vi "SPIDelaySet.vi"(8 "error in (no error)":errorcluster caption="错误输入（无错误）", 10 "Delay(CLK)":i32(ring) items=["0"=0, "1"=1, "2"=2, "5"=5, "10"=10, "20"=20], 11 "handle":u64) -> (0 "error out":errorcluster caption="错误输出", 2 "function return":i32, 3 "handle out":u64)   [LabVIEW 2018]
doc: "Set pos. or neg. Supply voltage"
uses:
  InstrumentsPlayground.lvlib
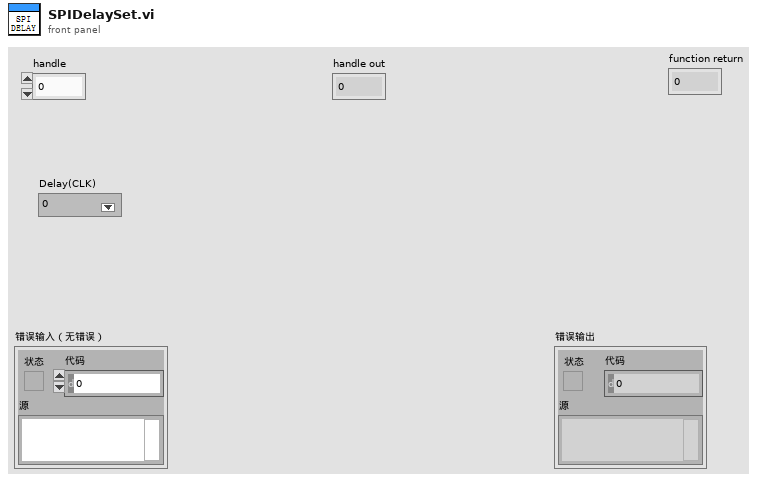
[diagram p1: front panel]
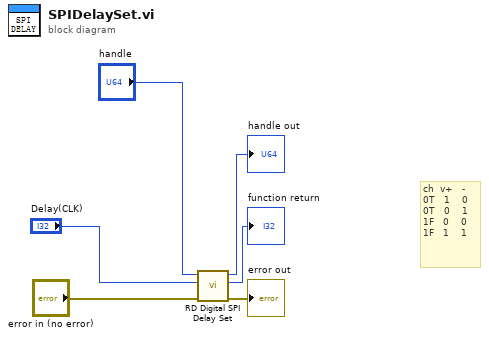
[diagram p0: block diagram]
diagram:
  # "ch  v+   -\n0T   1    0\n0T   0    1\n1F   0    0\n1F   1    1"
  n1 = call "RD Digital SPI Delay Set.vi"("error in (no error)"="error in (no error)", "delay"="Delay(CLK)", "handle"="handle") -> ("error out"=→"error out":errorcluster, "function return"=→"function return":i32, "handle out"=→"handle out":u64)  [unwired: 6 in]
